vi "Find Text Origin.vi"(9 "alignment(left, top)":T1, 10 "Bounding Rectangle":T2) -> (2 "origin(0,0)":cluster{"horizontal":i16, "vertical":i16})   [LabVIEW 2012, in "String XControl.xctl"]
uses:
  String XControl.xctl
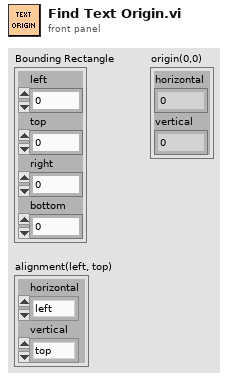
[diagram p1: front panel]
types:
  T1 = cluster{"horizontal":enum16{"left", "center", "right"}, "vertical":enum16{"top", "center", "bottom"}}
  T2 = cluster{"left":i16, "top":i16, "right":i16, "bottom":i16}
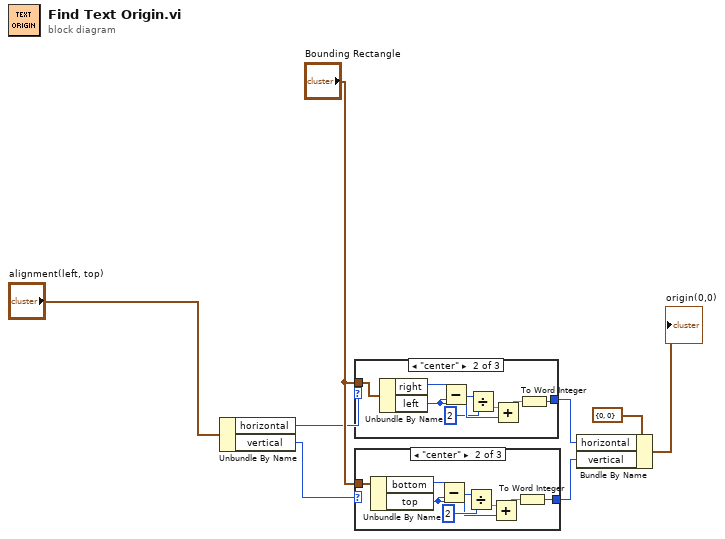
[diagram p0: block diagram]
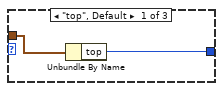
[diagram p2: hidden frame]
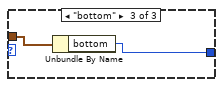
[diagram p3: hidden frame]
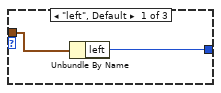
[diagram p4: hidden frame]
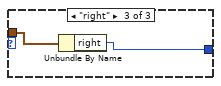
[diagram p5: hidden frame]
diagram:
  n1 = Unbundle By Name("alignment(left, top)") -> ("horizontal"=w2:enum16{"left", "center", "right"}, "vertical"=w3:enum16{"top", "center", "bottom"})
  n2 = case shown="\"center\"" w2 {
    tunnel: "Bounding Rectangle" -> [w10 w12 w20]
    tunnel: [w9 w11 w19] -> w6
    frame "left", Default {
      n3 = Unbundle By Name(w10) -> ("left"=w9:i16)
    }
    frame "center" {
      n4 = Unbundle By Name(w12) -> ("right"=w13:i16, "left"=w17:i16)
      n5 = Subtract(x=w13, y=w17) -> (x-y=w14:i16)
      n6 = Divide(x=w14, y=i16 2) -> (x/y=w16:dbl)
      n7 = Add(x=w16, y=w17) -> (x+y=w18:dbl)
      n8 = To Word Integer(number=w18) -> (16bit integer=w11:i16)
    }
    frame "right" {
      n9 = Unbundle By Name(w20) -> ("right"=w19:i16)
    }
  }
  n10 = case shown="\"center\"" w3 {
    tunnel: "Bounding Rectangle" -> [w22 w30 w32]
    tunnel: [w21 w23 w31] -> w7
    frame "top", Default {
      n11 = Unbundle By Name(w22) -> ("top"=w21:i16)
    }
    frame "center" {
      n12 = Unbundle By Name(w30) -> ("bottom"=w29:i16, "top"=w25:i16)
      n13 = Subtract(x=w29, y=w25) -> (x-y=w28:i16)
      n14 = Divide(x=w28, y=i16 2) -> (x/y=w26:dbl)
      n15 = Add(x=w26, y=w25) -> (x+y=w24:dbl)
      n16 = To Word Integer(number=w24) -> (16bit integer=w23:i16)
    }
    frame "bottom" {
      n17 = Unbundle By Name(w32) -> ("bottom"=w31:i16)
    }
  }
  n18 = Bundle By Name(cluster=cluster{"horizontal":i16, "vertical":i16} {"horizontal"=0, "vertical"=0} ("origin(0,0)"), "horizontal"=w6, "vertical"=w7) -> (→"origin(0,0)":cluster{"horizontal":i16, "vertical":i16})
